vi "Agilent VNA Read Channel Display.vi"(7 "Agilent VNA":T2, 8 "error in (no error)":errorcluster, 11 "VISA Resource Name":refnum<visa-resource-name>) -> (0 "error out":errorcluster, 2 "Display":T1, 3 "dup VISA Resource Name":refnum<visa-resource-name>)   [LabVIEW 2011]
uses:
  TypeDefs/Agilent VNA Display.ctl
  TypeDefs/Agilent VNA Instrument Info.ctl
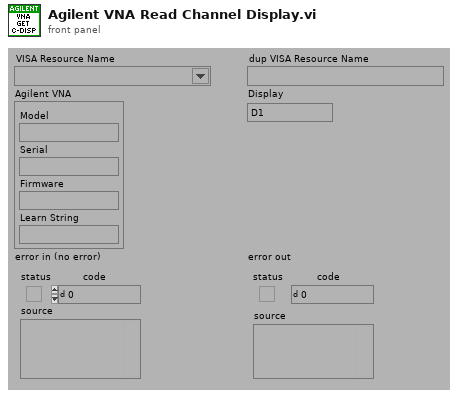
[diagram p1: front panel]
types:
  T1 = typedef "Agilent VNA Display.ctl" = enum16{"D1", "D12", "D1_2", "D112", "D1_1_2", "D123", "D1_2_3", "D12_33", "D11_23", "D13_23", "D12_13", "D1234", "D1_2_3_4", "D12_34", "D123_456", "D12_34_56", "D1234_5678", "D12_34_56_78", "D123_456_789", "D123__ABC", "D1234__9ABC", "D1234__DEFG"}
  T2 = typedef "Agilent VNA Instrument Info.ctl" = cluster{"Model":string, "Serial":string, "Firmware":string, "Learn String":string}
  T3 = typedef "Agilent VNA Model.ctl" = enum16{"Not Supported", "8510X", "8719X", "8720X", "8722X", "8753X", "ENA", "PNA", "Field Fox"}
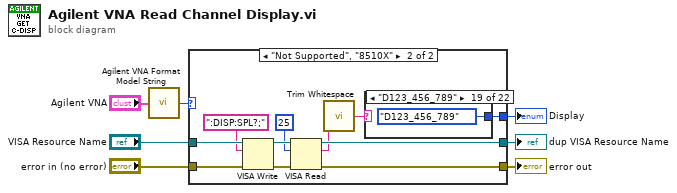
[diagram p0: block diagram]
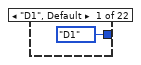
[diagram p3: hidden frame]
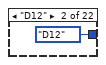
[diagram p4: hidden frame]
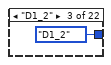
[diagram p5: hidden frame]
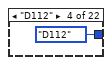
[diagram p6: hidden frame]
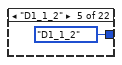
[diagram p7: hidden frame]
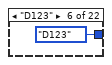
[diagram p8: hidden frame]
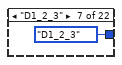
[diagram p9: hidden frame]
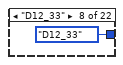
[diagram p10: hidden frame]
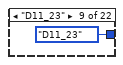
[diagram p11: hidden frame]
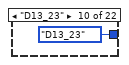
[diagram p12: hidden frame]
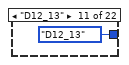
[diagram p13: hidden frame]
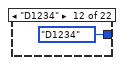
[diagram p14: hidden frame]
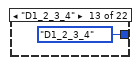
[diagram p15: hidden frame]
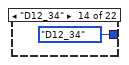
[diagram p16: hidden frame]
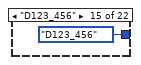
[diagram p17: hidden frame]
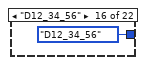
[diagram p18: hidden frame]
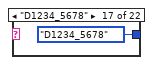
[diagram p19: hidden frame]
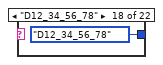
[diagram p20: hidden frame]
diagram:
  n1 = call "Agilent VNA Format Model String.vi"("Model"="Agilent VNA") -> ("Model"=w2:T3)
  n2 = case shown="\"E5070B\", \"E5071B\"" w2 {
    tunnel: "VISA Resource Name" -> [w9 w20]
    tunnel: "error in (no error)" -> [w8 w19]
    tunnel: [w9 w16] -> w5
    tunnel: [w8 w15] -> w4
    tunnel: [_ w10] -> w1
    frame Default {
    }
    frame "Not Supported", "8510X" {
      n3 = VISA Write(VISA resource name=w20, write buffer=":DISP:SPL?;", error in (no error)=w19) -> (VISA resource name out=w17:refnum<visa-resource-name>, error out=w18:errorcluster)  [unwired: 1 out]
      n4 = VISA Read(VISA resource name=w17, byte count=u32 25, error in (no error)=w18) -> (VISA resource name out=w16:refnum<visa-resource-name>, read buffer=w12:string, error out=w15:errorcluster)  [unwired: 1 out]
      n5 = call <vilib>:"Trim Whitespace.vi"("string"=w12) -> ("trimmed string"=w11:string)  [unwired: 1 in]
      n6 = case shown="\"D123_456_789\"" w11 {
        tunnel: [Agilent_VNA_Display."D1" ("Display") Agilent_VNA_Display."D12" ("Display") Agilent_VNA_Display."D1_2" ("Display") Agilent_VNA_Display."D112" ("Display") Agilent_VNA_Display."D1_1_2" ("Display") Agilent_VNA_Display."D123" ("Display") Agilent_VNA_Display."D1_2_3" ("Display") Agilent_VNA_Display."D12_33" ("Display") Agilent_VNA_Display."D11_23" ("Display") Agilent_VNA_Display."D13_23" ("Display") Agilent_VNA_Display."D12_13" ("Display") Agilent_VNA_Display."D1234" ("Display") Agilent_VNA_Display."D1_2_3_4" ("Display") Agilent_VNA_Display."D12_34" ("Display") Agilent_VNA_Display."D123_456" ("Display") Agilent_VNA_Display."D12_34_56" ("Display") Agilent_VNA_Display."D1234_5678" ("Display") Agilent_VNA_Display."D12_34_56_78" ("Display") Agilent_VNA_Display."D123_456_789" ("Display") Agilent_VNA_Display."D123__ABC" ("Display") Agilent_VNA_Display."D1234__9ABC" ("Display") Agilent_VNA_Display."D1234__DEFG" ("Display")] -> w10
        frame "D1", Default {
        }
        frame "D12" {
        }
        frame "D1_2" {
        }
        frame "D112" {
        }
        frame "D1_1_2" {
        }
        frame "D123" {
        }
        frame "D1_2_3" {
        }
        frame "D12_33" {
        }
        frame "D11_23" {
        }
        frame "D13_23" {
        }
        frame "D12_13" {
        }
        frame "D1234" {
        }
        frame "D1_2_3_4" {
        }
        frame "D12_34" {
        }
        frame "D123_456" {
        }
        frame "D12_34_56" {
        }
        frame "D1234_5678" {
        }
        frame "D12_34_56_78" {
        }
        frame "D123_456_789" {
        }
        frame "D123__ABC" {
        }
        frame "D1234_9ABC" {
        }
        frame "D1234_DEFG" {
        }
      }
    }
  }
  "dup VISA Resource Name" <- w5
  "error out" <- w4
  "Display" <- w1
